vi "All Tests.vi"   [LabVIEW 2021, in "Ring Buffer Strict Accessor Unit Tests.lvlib"]
uses:
  Ring Buffer Strict Accessor Unit Tests.lvlib
  <vilib>/addons/_JKI Toolkits/Caraya/run-tests/Run Test (Scalar Path).vi
  <vilib>/addons/_JKI Toolkits/Caraya/Caraya.lvlib
  <userlib>/_OpenG.lib/file/file.llb/openg_file.lvlib
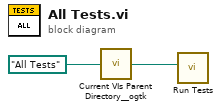
[diagram p0: block diagram]
diagram:
  n1 = call <userlib>:"Current VIs Parent Directory__ogtk.vi"("Relative path (.)"=path "All Tests" ("Test Path")) -> ("Parent Directory (+ Relative)"=w1:path)  [unwired: 4 in]
  n2 = call-poly <vilib>:"Run Tests.vi"("Test Path"=w1) -> ()  [unwired: 9 in, 2 out]
